vi "Write Data Type.vi"(8 "error in (no error)":errorcluster, 10 "Data Type":string, 11 "User Sender in":refnum<class "User Sender.lvclass">) -> (0 "error out":errorcluster, 3 "User Sender out":refnum<class "User Sender.lvclass">)   [LabVIEW 2023, in "User Sender.lvclass"]
uses:
  User Sender.lvclass
  User Sender.lvclass/User Sender.ctl
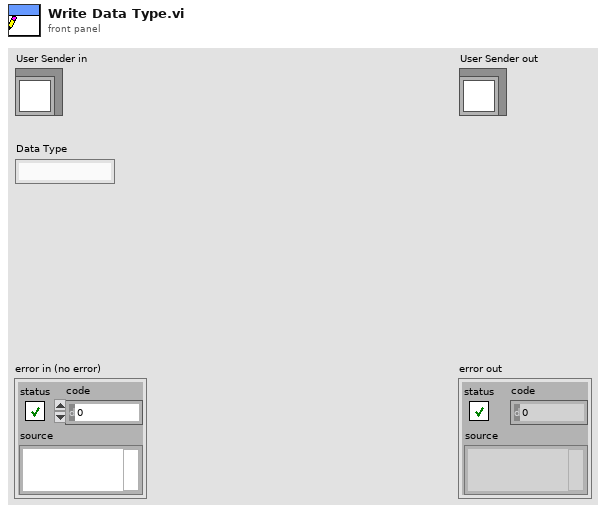
[diagram p1: front panel]
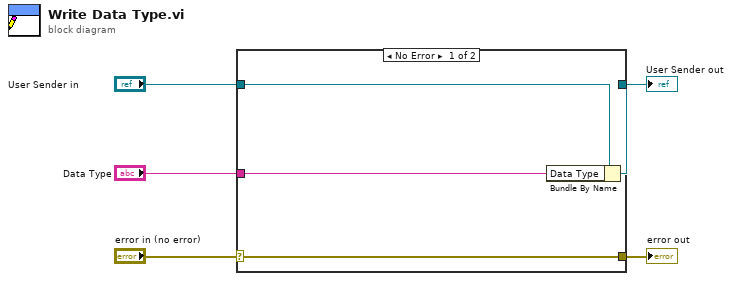
[diagram p0: block diagram]
diagram:
  n1 = case shown="No Error" "error in (no error)" {
    selector: "error in (no error)" -> [w9 w10]
    tunnel: [w9 w10] -> w4
    tunnel: [w7 w11] -> w2
    tunnel: "User Sender in" -> [w8 w11]
    tunnel: "Data Type" -> [w6 _]
    frame No Error {
      n2 = Bundle By Name(cluster=w8, "Data Type"=w6) -> (w7:refnum<class "User Sender.lvclass">)
    }
    frame Error {
    }
  }
  "error out" <- w4
  "User Sender out" <- w2
